vi "Asynchronous Stream 4310 DMM.vi"(10 "Sample Rate":i32=20000, 11 "gRPCid":T1) -> ()   [LabVIEW 2019]
uses:
  VIs/grpcId.ctl
  Global Operations.ctl
  VIs/gprc-support.lvlib
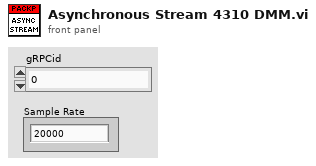
[diagram p1: front panel]
types:
  T1 = typedef "gprc-support.lvlib/grpcId.ctl" = u64
  T2 = typedef "Global Operations.ctl" = enum16{"Get", "Set"}
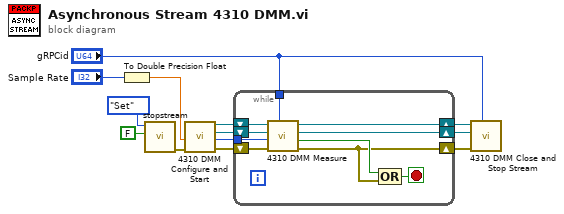
[diagram p0: block diagram]
diagram:
  n1 = To Double Precision Float(number="Sample Rate") -> (double precision float=w1:dbl)
  n2 = call "stopstream.vi"("STOPSTREAM"=FALSE, "Operation"=Global_Operations."Set") -> ("error out"=w6:errorcluster)  [unwired: 8 in, 1 out]
  n3 = call "4310 DMM Configure and Start.vi"("Sample Rate"=w1, "error in (no error)"=w6) -> ("IVI Refnum out"=w7:refnum<k15>, "task out"=w8:refnum<k21>, "Number of Samples out"=w9:i32, "error out"=w10:errorcluster)  [unwired: 14 in]
  n4 = while {
    tunnel: w9 -> [w21]
    shift-right: [w19] -> w11
    shift-left: w7 -> [w23]
    shift-right: [w18] -> w12
    shift-left: w8 -> [w22]
    shift-right: [w14] -> w13
    shift-left: w10 -> [w20]
    tunnel: "gRPCid" -> [w17]
    stop <- w16 stop-if-true
    n5 = call "4310 DMM Measure.vi"("IVI Refnum in"=w23, "task in"=w22, "Number of Samples in"=w21, "error in"=w20, "gRPCid"=w17) -> ("IVI Refnum out"=w19:refnum<k15>, "task out"=w18:refnum<k21>, "STOPSTREAM?"=w15:bool, "error out"=w14:errorcluster)  [unwired: 2 in]
    n6 = Compound Arithmetic op=OR(w15, w14) -> (w16:bool)
  }
  n7 = call "4310 DMM Close and Stop Stream.vi"("gRPCid"="gRPCid", "error in (no error)"=w13, "task in"=w12, "IVI Refnum in"=w11) -> ()  [unwired: 7 in, 1 out]
